vi "AlliGator Best of All (weights) String.vi"(1 "Weights":T1 caption="Weighted Fit") -> (0 "Weights String":string caption="Weighted Fit")   [LabVIEW 2021, in "AlliGator Decay Analysis.lvlib" / "AlliGator Decay Fit.lvlib"]
doc: "String to append to the fit output sent to the Notebook in the case of a \"Best of All\" option, to specify which fit was the best (weighted or unweighted)."
uses:
  Fits/IRF(X)PSED/Fit Weights Type.ctl
  AlliGator Decay Fit.lvlib
  Fits/Fits.lvlib
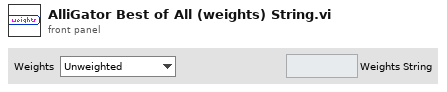
[diagram p1: front panel]
types:
  T1 = typedef "Fits.lvlib/Fit Weights Type.ctl" = enum16{"Unweighted", "1/Variance", "Best of All"}
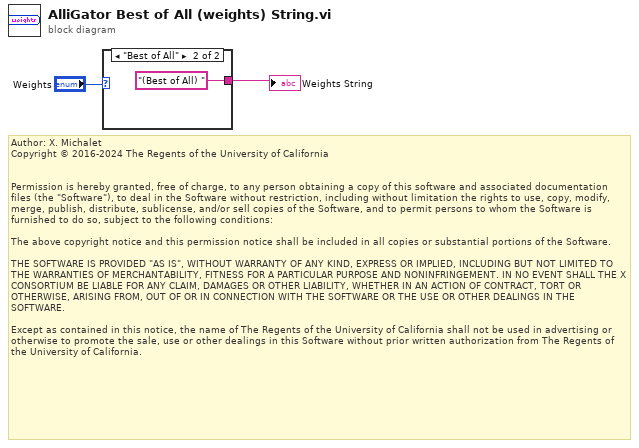
[diagram p0: block diagram]
diagram:
  # "Author: X. Michalet\nCopyright © 2016-2024 The Regents of the University of California\n \n\nPermission is hereby granted, free of charge, to any person obtaining a copy of this software and associated documentation files (the \"Software\"), to deal in the Software without restriction, including without limitation the rights to use, copy, modify, merge, publish, distribute, sublicense, and/or sell copies of the Software, and to permit persons to whom the Software is furnished to do so, subject to the following conditions:\n\nThe above copyright notice and this permission notice shall be included in all copies or substantial portions of the Software.\n\nTHE SOFTWARE IS PROVIDED \"AS IS\", WITHOUT WARRANTY OF ANY KIND, EXPRESS OR IMPLIED, INCLUDING BUT NOT LIMITED TO THE WARRANTIES OF MERCHANTABILITY, FITNESS FOR A PARTICULAR PURPOSE AND NONINFRINGEMENT. IN NO EVENT SHALL THE X CONSORTIUM BE LIABLE FOR ANY CLAIM, DAMAGES OR OTHER LIABILITY, WHETHER IN AN ACTION OF CONTRACT, TORT OR OTHERWISE, ARISING FROM, OUT OF OR IN CONNECTION WITH THE SOFTWARE OR THE USE OR OTHER DEALINGS IN THE SOFTWARE.\n\nExcept as contained in this notice, the name of The Regents of the University of California shall not be used in advertising or otherwise to promote the sale, use or other dealings in this Software without prior written authorization from The Regents of the University of California."
  n1 = case shown="\"Best of All\"" "Weights" {
    tunnel: [_ "(Best of All) " ("Weights String")] -> w1
    frame "Unweighted", Default {
    }
    frame "Best of All" {
    }
  }
  "Weights String" <- w1
